vi "io(1).vi"() -> ()   [LabVIEW 2018]
uses:
  Global_variables.vi
  <vilib>/Instr/_visa.llb/VISA Configure Serial Port (Instr).vi
panel:
  out "滑动杆 2":dbl(slide) scale=0.0..2.0
  out "Error Out":errorcluster caption="错误输出"
  out "TEST_P_PWM":dbl
  out "TEST_A_PWM":dbl
  out "PWML":u16
  out "PWMH":u16
  out "滑动杆":dbl(slide) scale=-7200.0..7200.0
  out "ENCM":u8
  out "返回数":u32
  out "PWM":dbl
  out "read buffer":string
  out "ADC":u16
  out "Encoder":u16
  out "ENCL":u8
  out "ENCH":u8
  out "ADCL":u8
  out "ADCH":u8
  in  "读取":bool
  in  "读数":u32=1000
  out "最大误差":dbl[](array[numeric])
  out "字符串":string
  in  "自动起摆        手动起摆":bool
  out "累计误差":dbl[](array[numeric])
  in  "On/Off":bool
  in  "VISA resource name":refnum<visa-resource-name> caption="VISA资源名称"
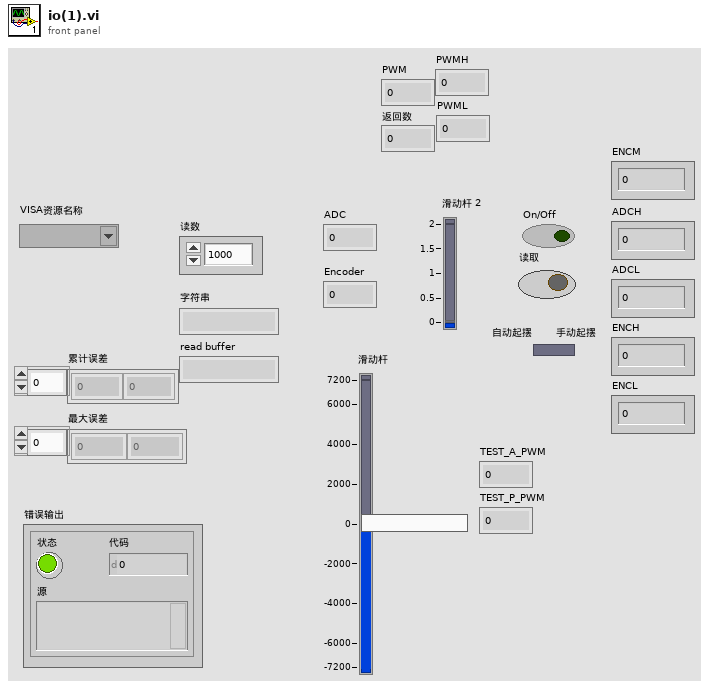
[diagram p1: front panel]
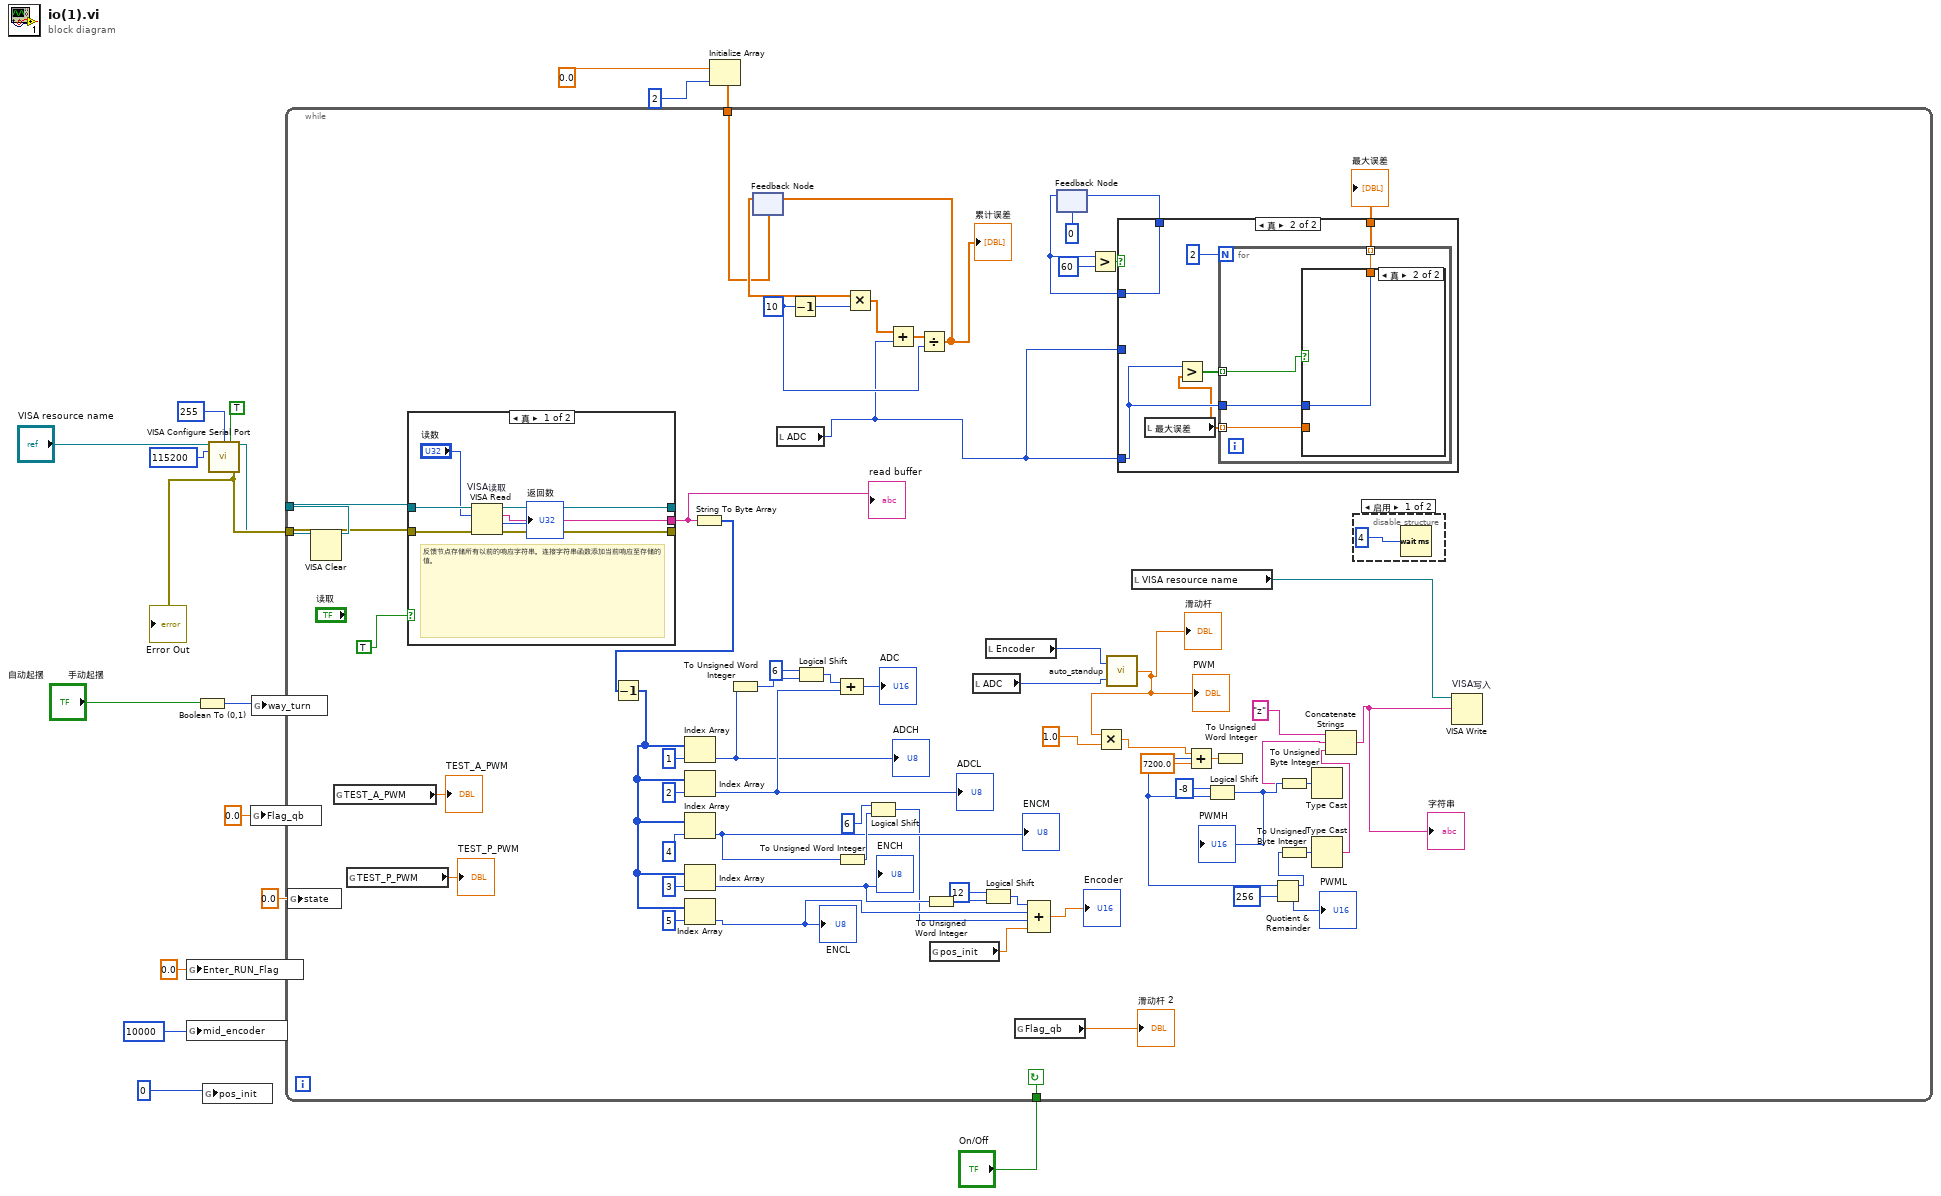
[diagram p0: block diagram]
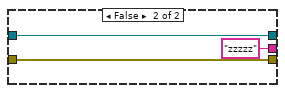
[diagram p2: hidden frame]
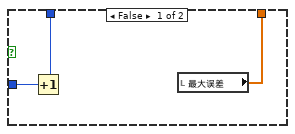
[diagram p4: hidden frame]
diagram:
  n1 = global write "Global_variables.vi" "Enter_RUN_Flag"(0.0 ("Enter_RUN_Flag")) -> ()
  n2 = global write "Global_variables.vi" "mid_encoder"(10000) -> ()
  n3 = Boolean To (0,1)(Boolean="自动起摆        手动起摆") -> (0, 1=w11:i16)
  n4 = global write "Global_variables.vi" "pos_init"(0) -> ()
  n5 = call-poly "VISA Configure Serial Port"("VISA resource name"="VISA resource name", "termination char\n(0xA = '\\n' = LF)"=u8 255 ("termination char\n(0xA = '\\n' = LF)"), "Enable Termination\nChar (T)"=TRUE ("Enable Termination\nChar (T)"), "baud rate (9600)"=u32 115200) -> ("VISA resource name out"=w2:refnum<visa-resource-name>, "error out"=w5:errorcluster)  [unwired: 10 in]
  "Error Out" <- w5
  n6 = global write "Global_variables.vi" "Flag_qb"(0.0 ("Flag_qb")) -> ()
  n7 = global write "Global_variables.vi" "way_turn"(w11) -> ()
  n8 = global write "Global_variables.vi" "state"(0.0 ("state")) -> ()
  n9 = VISA Clear(VISA resource name=w2) -> (VISA resource name out=w3:refnum<visa-resource-name>)  [unwired: 1 in, 1 out]
  n10 = Initialize Array(0.0 ("元素"), 2 ("维数大小")) -> (w12:dbl[])
  n11 = while {
    tunnel: w3 -> [w68]
    tunnel: w5 -> [w67]
    tunnel: "On/Off" -> [w83]
    tunnel: w12 -> [w76]
    stop <- w83 continue-if-true
    w77 = 10
    n12 = global read "Global_variables.vi" "TEST_A_PWM"() -> (→"TEST_A_PWM":dbl)
    n13 = global read "Global_variables.vi" "TEST_P_PWM"() -> (→"TEST_P_PWM":dbl)
    n14 = case shown="真" TRUE {
      tunnel: [w88 w93] -> _
      tunnel: w68 -> [w90 w93]
      tunnel: [w86 w92] -> _
      tunnel: w67 -> [w89 w92]
      tunnel: [w85 "zzzzz" ("read buffer")] -> w19
      frame True {
        # "反馈节点存储所有以前的响应字符串。连接字符串函数添加当前响应至存储的值。"
        n15 = VISA Read "VISA读取"(VISA resource name=w90, byte count="读数", error in (no error)=w89) -> (VISA resource name out=w88:refnum<visa-resource-name>, read buffer=w85:string, return count=→"返回数":u32, error out=w86:errorcluster)
      }
      frame False {
      }
    }
    "read buffer" <- w19
    n16 = String To Byte Array(string=w19) -> (unsigned byte array=w39:u8[])
    n17 = Decrement(x=w39) -> (x-1=w38:u8[])
    n18 = Index Array(array=w38, index=1 ("索引")) -> (element=w43:u8)
    "ADCH" <- w43
    n19 = Index Array(array=w38, index=2 ("索引")) -> (element=w44:u8)
    "ADCL" <- w44
    n20 = Index Array(array=w38, index=4 ("索引")) -> (element=w41:u8)
    "ENCM" <- w41
    n21 = Index Array(array=w38, index=3 ("索引")) -> (element=w63:u8)
    "ENCH" <- w63
    n22 = Index Array(array=w38, index=5 ("索引")) -> (element=w60:u8)
    "ENCL" <- w60
    n23 = To Unsigned Word Integer(number=w43) -> (unsigned 16bit integer=w55:u16)
    n24 = feedback #1(w76) -> (w81:dbl[])
    n25 = local read "ADC"() -> (w51:u16)
    n26 = Decrement(x=w77) -> (x-1=w82:i32)
    n27 = Logical Shift(y=i16 6, x=w55) -> (x << y=w56:u16)
    n28 = To Unsigned Word Integer(number=w41) -> (unsigned 16bit integer=w45:u16)
    n29 = Compound Arithmetic op=unknown(w56, w44) -> (→"ADC":u16)
    n30 = Multiply(x=w81, y=w82) -> (x*y=w80:dbl[])
    n31 = Logical Shift(y=i16 6, x=w45) -> (x << y=w40:u16)
    n32 = Add(x=w80, y=w51) -> (x+y=w78:dbl[])
    n33 = Divide(x=w78, y=w77) -> (x/y=w79:dbl[])
    "累计误差" <- w79
    n34 = feedback-in #1(w79) -> ()
    n35 = To Unsigned Word Integer(number=w63) -> (unsigned 16bit integer=w62:u16)
    n36 = global read "Global_variables.vi" "pos_init"() -> (w20:dbl)
    n37 = local read "ADC"() -> (w53:u16)
    n38 = Logical Shift(y=i16 12, x=w62) -> (x << y=w59:u16)
    n39 = local read "Encoder"() -> (w52:u16)
    n40 = global read "Global_variables.vi" "Flag_qb"() -> (→"滑动杆 2":dbl)
    n41 = Compound Arithmetic op=ADD(w59, w60, w40, w20) -> (→"Encoder":dbl)
    n42 = feedback #2(0) -> (w71:i32)
    n43 = Greater?(x=w71, y=60) -> (0:w73:bool)
    n44 = call "auto_standup.vi"("Angle"=w53, "Encoder"=w52) -> ("PWM"=w22:dbl)
    "PWM" <- w22
    "滑动杆" <- w22
    n45 = Multiply(x=w22, y=1.0) -> (x*y=w23:dbl)
    n46 = case shown="真" w73 {
      tunnel: w71 -> [w97 w103]
      tunnel: [w96 w103] -> w70
      tunnel: w51 -> [_ _]
      tunnel: w51 -> [_ w100]
      tunnel: [w95 w99] -> w69
      frame False {
        n47 = Increment(x=w97) -> (x+1=w96:i32)
        n48 = local read "最大误差"() -> (w95:dbl[])
      }
      frame True {
        n49 = local read "最大误差"() -> (w98:dbl[])
        n50 = Greater?(x=w100, y=w98) -> (0:w101:bool[])
        n51 = for {
          N: 2 -> [_]
          tunnel: w101 -> [w107] mode=indexing
          tunnel: w100 -> [w106]
          tunnel: [w105] -> w99 mode=indexing
          tunnel: w98 -> [w104] mode=indexing
          n52 = case shown="真" w107 {
            tunnel: w106 -> [_ w109]
            tunnel: [w108 w109] -> w105
            tunnel: w104 -> [w108 _]
            frame False {
            }
            frame True {
            }
          }
        }
      }
    }
    "最大误差" <- w69
    n53 = feedback-in #2(w70) -> ()
    n54 = local read "VISA resource name"() -> (w75:refnum<visa-resource-name>)
    n55 = Add(x=w23, y=7200.0) -> (x+y=w37:dbl)
    n56 = To Unsigned Word Integer(number=w37) -> (unsigned 16bit integer=w32:u16)
    n57 = Logical Shift(y=i16 -8, x=w32) -> (x << y=w34:u16)
    "PWMH" <- w34
    n58 = Quotient & Remainder(x=w32, y=u16 256) -> (x-y*floor(x/y)=w29:u16)  [unwired: 1 out]
    "PWML" <- w29
    n59 = To Unsigned Byte Integer(number=w34) -> (unsigned 8bit integer=w36:u8)
    n60 = To Unsigned Byte Integer(number=w29) -> (unsigned 8bit integer=w30:u8)
    n61 = Type Cast(x=w36) -> (*(type *) &x=w33:string)  [unwired: 1 in]
    n62 = Type Cast(x=w30) -> (*(type *) &x=w28:string)  [unwired: 1 in]
    n63 = Concatenate Strings("z" ("字符串"), w33, w28) -> (w47:string)
    "字符串" <- w47
    n64 = disable-structure shown="启用" {
      frame Enabled {
        n65 = Wait (ms)(milliseconds to wait=4) -> ()  [unwired: 1 out]
      }
      frame Disabled {
      }
    }
    n66 = VISA Write "VISA写入"(VISA resource name=w75, write buffer=w47) -> ()  [unwired: 1 in, 3 out]
  }
